vi "FPGA_target_read_fifo.vi"(6 "data_in":T1, 8 "read_fifo":bool, 9 "C1_in":T2) -> (10 "fifo_empty":bool, 12 "data_out":T1, 13 "C1_out":T2)   [LabVIEW 2014]
doc: "Reads new data from the internal FIFO (or pipes the old data through)"
uses:
  FPGA_32BitPattern_data_type.ctl
  FPGA_cmd_data_type.ctl
  <vilib>/rvi/eio/common/nirviEmuReportErrorAndStop.vi
  <vilib>/rvi/errors/nirviReportUnexpectedCaseInternalError.vi
  <vilib>/rvi/errors/nirviReportUnexpectedCaseInternalError (U32).vi
  <vilib>/rvi/Emulation/niFpgaProcessEmulError.vi
  <vilib>/rvi/occurrence/nirviWaitOnOccurrenceBase.vi
  <vilib>/rvi/FIFO/Fifo_Resource/nirvififoEmulationReleaseLock.vi
  <vilib>/rvi/FIFO/Fifo_Resource/nirvififoEmulationObtainLock.vi
  <vilib>/rvi/FIFO/Fifo_Resource/nirvififoEmulationCreateLock.vi
  <vilib>/rvi/DataTransferAndStorage/Container/Common/niFpgaContainerGetUniqueNameForEmu.vi
  <vilib>/rvi/FIFO/Fifo_Resource/nirvififoEmulationSetSize.vi
  <vilib>/rvi/FIFO/Fifo_Resource/nirviFifoEmulationQueueMgr.vi
  <instcachedir>/0/nirviFifoEmulationQueueMgr_E5CAEC123FF24DC58D834DCA3CDAA9B5.lvgen/nirviFifoEmulationQueueMgr_E5CAEC123FF24DC58D834DCA3CDAA9B5_002.vi
  <vilib>/rvi/errors/niFpgaSetErrorForExecOnDevCompSimple.vi
  <vilib>/rvi/Emulation/niFpgaSctlEmulationGetInTimedLoop.vi
  <vilib>/rvi/Emulation/niFpgaEmulationIsFPGAContextNoSignature.vi
  <instcachedir>/0/nirviFifoEmulationQueueMgr_E5CAEC123FF24DC58D834DCA3CDAA9B5.lvgen/nirviFifoEmulationQueueMgr_E5CAEC123FF24DC58D834DCA3CDAA9B5_003.vi
  <instcachedir>/0/nirviFifoEmulationQueueMgr_E5CAEC123FF24DC58D834DCA3CDAA9B5.lvgen/nirviFifoEmulationQueueMgr_E5CAEC123FF24DC58D834DCA3CDAA9B5_001.vi
  <vilib>/rvi/DataTransferAndStorage/Container/XNode/niFpgaContainer.xnode
  <vilib>/rvi/FIFO/Fifo_Resource/nirvififoEmulationRead.vi
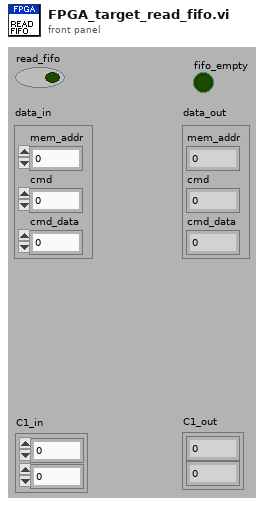
[diagram p1: front panel]
types:
  T1 = typedef "FPGA_cmd_data_type.ctl" = cluster{"mem_addr":u32, "cmd":u8, "cmd_data":u32}
  T2 = typedef "FPGA_32BitPattern_data_type.ctl" = cluster{"port0":u8, "port1":u8}
  T3 = cluster{"Element":u32, "Element":u8, "Element":u32}
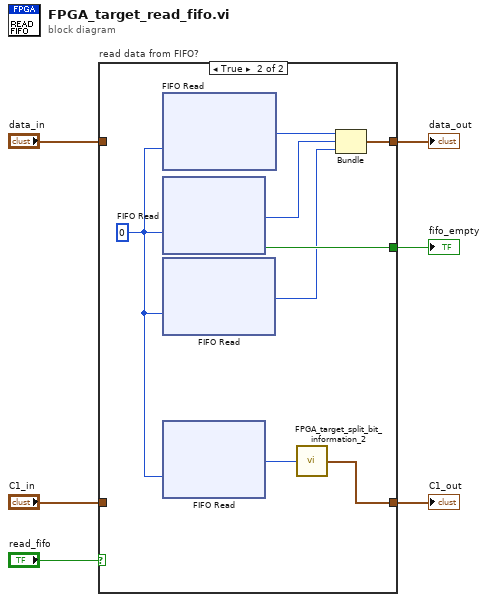
[diagram p0: block diagram]
diagram:
  n1 = case "read data from FIFO?" shown="True" "read_fifo" {
    selector: "read_fifo" -> [w8 _]
    tunnel: [w8 w17] -> w6
    tunnel: [w9 w15] -> w4
    tunnel: "C1_in" -> [w9 _]
    tunnel: "data_in" -> [w7 _]
    tunnel: [w7 w14] -> w1
    frame False {
    }
    frame True {
      w10 = 0 ("Timeout")
      n2 = xnode ("FIFO Read")("Timeout"=w10) -> ("Element"=w11:u32)  [unwired: 1 in, 2 out]
      n3 = xnode ("FIFO Read")("Timeout"=w10) -> ("Element"=w13:u8, "Timed Out?"=w17:bool)  [unwired: 1 in, 1 out]
      n4 = xnode ("FIFO Read")("Timeout"=w10) -> ("Element"=w12:u32)  [unwired: 1 in, 2 out]
      n5 = xnode ("FIFO Read")("Timeout"=w10) -> ("Element"=w16:u16)  [unwired: 1 in, 2 out]
      n6 = call "FPGA_target_split_bit_information_2.vi"("data in"=w16) -> ("connector_data"=w15:T2)
      n7 = Bundle("Element"=w11, "Element"=w13, "Element"=w12) -> (w14:T3)  [unwired: 1 in]
    }
  }
  "fifo_empty" <- w6
  "C1_out" <- w4
  "data_out" <- w1
